vi "Append Watermark polymorphic.vi"   [LabVIEW 2012]
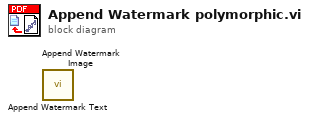
[diagram p0: block diagram]
diagram:
  n1 = call "Append Watermark Text.vi"() -> ()  [unwired: 14 in, 2 out]
  n2 = call "Append Watermark Image.vi"() -> ()  [unwired: 14 in, 2 out]
